vi "SubVI_RandomiseMatrix.vi"(8 "Y":dbl[](array[numeric]), 11 "X":dbl[](array[numeric])) -> (0 "N":i32, 1 "Random index":i32[](array[numeric]), 2 "Y shuffled":dbl[](array[numeric]), 3 "X shuffled":dbl[](array[numeric]))   [LabVIEW 2019]
uses:
  <vilib>/Analysis/1siggen.llb/Riffle Array (DBL).vi
  <vilib>/Analysis/NI_AALBase.lvlib
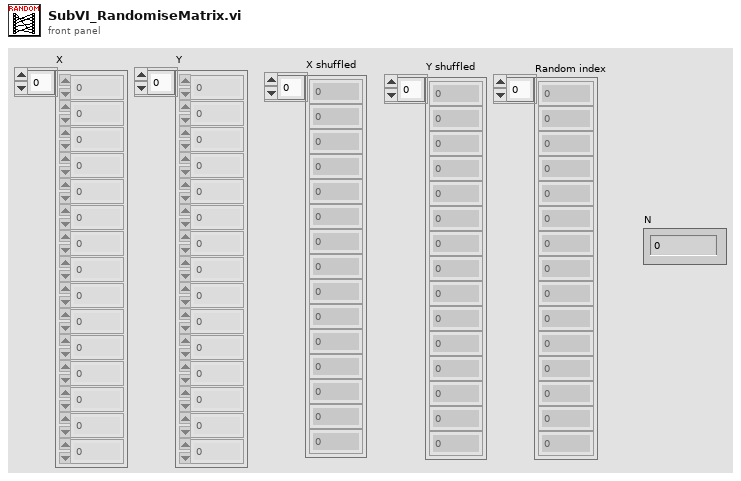
[diagram p1: front panel]
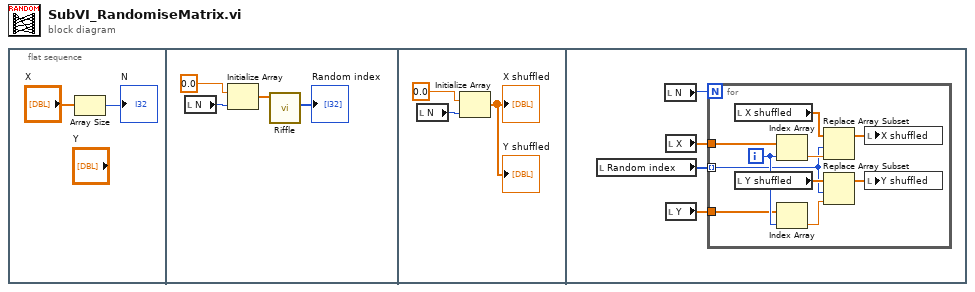
[diagram p0: block diagram]
diagram:
  n1 = flat-sequence {
    frame #0 {
      n2 = Array Size(array="X") -> (size(s)=→"N":i32)
    }
    frame #1 {
      n3 = local read "N"() -> (w6:i32)
      n4 = Initialize Array(0.0 ("element"), w6) -> (w4:dbl[])
      n5 = call-poly <vilib>:"Riffle.vi"("X"=w4) -> ("Riffled Index"=→"Random index":i32[])  [unwired: 8 in, 2 out]
    }
    frame #2 {
      n6 = local read "N"() -> (w8:i32)
      n7 = Initialize Array(0.0, w8) -> (→"X shuffled" →"Y shuffled":dbl[])
    }
    frame #3 {
      n8 = local read "Random index"() -> (w10:i32[])
      n9 = local read "N"() -> (w13:i32)
      n10 = local read "X"() -> (w12:dbl[])
      n11 = local read "Y"() -> (w11:dbl[])
      n12 = for {
        N: w13 -> [_]
        tunnel: w12 -> [w18]
        tunnel: w11 -> [w17]
        tunnel: w10 -> [w14] mode=indexing
        i -> [w19]
        n13 = local read "X shuffled"() -> (w21:dbl[])
        n14 = local read "Y shuffled"() -> (w23:dbl[])
        n15 = Index Array(array=w18, index=w19) -> (element=w15:dbl)
        n16 = Index Array(array=w17, index=w19) -> (element=w16:dbl)
        n17 = Replace Array Subset(array=w21, new element=w15, index=w14) -> (w20:dbl[])
        n18 = Replace Array Subset(array=w23, new element=w16, index=w14) -> (w22:dbl[])
        n19 = local write "X shuffled"(w20) -> ()
        n20 = local write "Y shuffled"(w22) -> ()
      }
    }
  }
